vi "AcqType.vi"(11 "Ch & spans + mod limits":T2[](array[typedef]) {"low limit (-10V)" format="%.3f"; "high limit (10V)" format="%.3f"}) -> (0 "cDAQ i":i32[](array[numeric]), 1 "eDAQ i":i32[][](array[numeric]), 2 "cDAQ tasks":refnum<k21>[](array[refnum]), 3 "eDAQ tasks":refnum<k21>[](array[refnum]), 4 "PXI i":i32[](array[numeric]), 5 "PXIs":refnum<k21>[](array[refnum]))   [LabVIEW 2013]
doc: "Figures out if the channels requested are cDAQ, eDAQ or PXI and whether eDAQ channels are over multiple chassis.\n\n#optimation"
uses:
  Controls/Ch_and_Spans.ctl
  Channels_and_Index.ctl
panel:
  out "cDAQs":T1[][](array[typedef])
  out "PXI":T1[](array[typedef])
  out "Number of cDAQs":i32
  out "eDAQs":T1[][](array[typedef])
  out "Number of eDAQs":i32
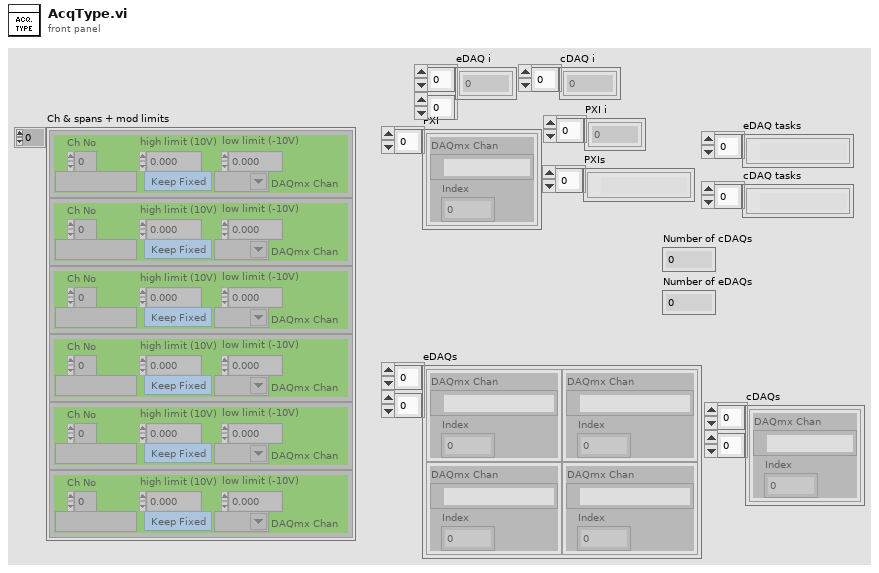
[diagram p1: front panel]
types:
  T1 = typedef "Channels_and_Index.ctl" = cluster{"DAQmx Chan":tag, "Index":i32}
  T2 = typedef "Ch_and_Spans.ctl" = cluster{"high limit (10V)":sgl, "low limit (-10V)":sgl, "Ch No":i16, "Var name":string, "Use Latest Calib":bool, "DAQmx Chan":tag}
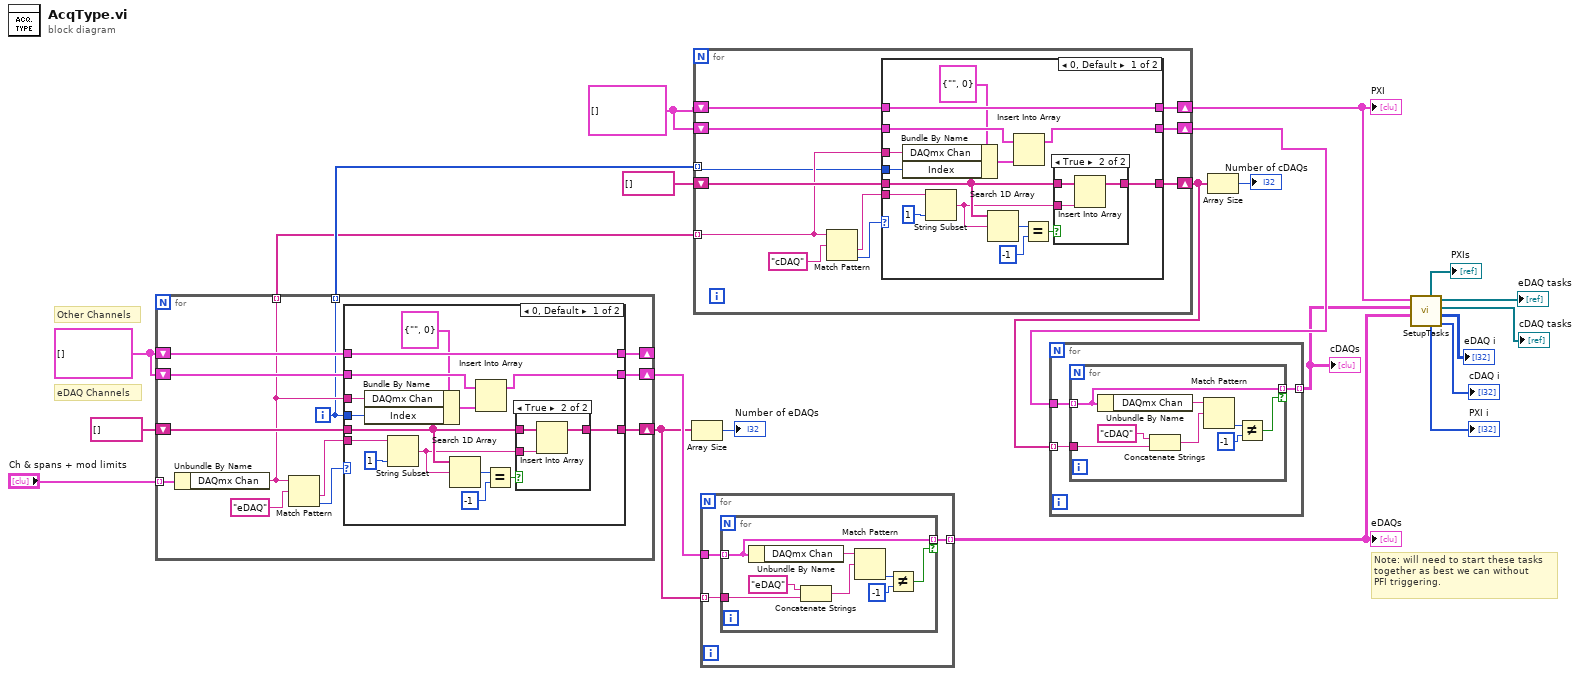
[diagram p0: block diagram]
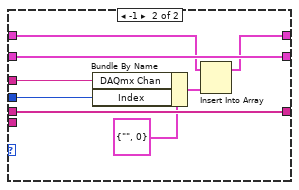
[diagram p3: hidden frame]
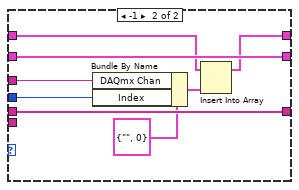
[diagram p5: hidden frame]
diagram:
  w15 = T1[] []
  w19 = T1[] []
  # "Note: will need to start these tasks \ntogether as best we can without\nPFI triggering."
  # "eDAQ Channels"
  # "Other Channels"
  n1 = for {
    tunnel: "Ch & spans + mod limits" -> [w34] mode=indexing
    shift-right: [w29] -> _
    shift-left: w19 -> [w31]
    shift-right: [w28] -> w18
    shift-left: w19 -> [w30]
    shift-right: [w25] -> w17
    shift-left: string[] [] -> [w27]
    tunnel: [w24] -> w3 mode=indexing
    tunnel: [w23] -> w4 mode=indexing
    i -> [w23]
    n2 = Unbundle By Name(w34) -> ("DAQmx Chan"=w24:tag)
    n3 = Match Pattern(string=w24, regular expression="eDAQ") -> (after substring=w26:string, offset past match=w32:i32)  [unwired: 1 in, 2 out]
    n4 = case shown="0, Default" w32 {
      tunnel: w24 -> [w36 w55]
      tunnel: w31 -> [w49 w60]
      tunnel: w30 -> [w48 w61]
      tunnel: [w49 w59] -> w29
      tunnel: [w47 w61] -> w28
      tunnel: w27 -> [w43 w58]
      tunnel: w26 -> [w45 _]
      tunnel: [w44 w58] -> w25
      tunnel: w23 -> [w35 w54]
      frame 0, Default {
        n5 = Bundle By Name(cluster=T1 {"DAQmx Chan"="", "Index"=0} ("Indexes"), "DAQmx Chan"=w36, "Index"=w35) -> (w37:T1)
        n6 = String Subset(string=w45, length (rest)=1 ("length (rest)")) -> (substring=w42:string)  [unwired: 1 in]
        n7 = Search 1D Array(1D array=w43, element=w42) -> (index of element=w41:i32)  [unwired: 1 in]
        n8 = Insert Into Array(array=w48, new element=w37) -> (w47:T1[])  [unwired: 1 in]
        n9 = Equal?(x=w41, y=-1) -> (x = y?=w39:bool)
        n10 = case shown="True" w39 {
          tunnel: [w50 w53] -> w44
          tunnel: w43 -> [w50 w52]
          tunnel: w42 -> [_ w51]
          frame False {
          }
          frame True {
            n11 = Insert Into Array(array=w52, new element=w51) -> (w53:string[])  [unwired: 1 in]
          }
        }
      }
      frame -1 {
        n12 = Bundle By Name(cluster=T1 {"DAQmx Chan"="", "Index"=0} ("Indexes"), "DAQmx Chan"=w55, "Index"=w54) -> (w56:T1)
        n13 = Insert Into Array(array=w60, new element=w56) -> (w59:T1[])  [unwired: 1 in]
      }
    }
  }
  n14 = Array Size(array=w17) -> (size(s)=→"Number of eDAQs":i32)
  n15 = for {
    shift-right: [w68] -> w13
    shift-left: w15 -> [w70]
    shift-right: [w67] -> w8
    shift-left: w15 -> [w69]
    shift-right: [w64] -> w9
    shift-left: string[] [] -> [w66]
    tunnel: w4 -> [w62] mode=indexing
    tunnel: w3 -> [w63] mode=indexing
    n16 = Match Pattern(string=w63, regular expression="cDAQ") -> (after substring=w65:string, offset past match=w71:i32)  [unwired: 1 in, 2 out]
    n17 = case shown="0, Default" w71 {
      tunnel: w63 -> [w74 w93]
      tunnel: w70 -> [w87 w98]
      tunnel: w69 -> [w86 w99]
      tunnel: [w87 w97] -> w68
      tunnel: [w85 w99] -> w67
      tunnel: w66 -> [w81 w96]
      tunnel: w65 -> [w83 _]
      tunnel: [w82 w96] -> w64
      tunnel: w62 -> [w73 w92]
      frame 0, Default {
        n18 = Bundle By Name(cluster=T1 {"DAQmx Chan"="", "Index"=0} ("Indexes"), "DAQmx Chan"=w74, "Index"=w73) -> (w75:T1)
        n19 = String Subset(string=w83, length (rest)=1 ("length (rest)")) -> (substring=w80:string)  [unwired: 1 in]
        n20 = Search 1D Array(1D array=w81, element=w80) -> (index of element=w79:i32)  [unwired: 1 in]
        n21 = Insert Into Array(array=w86, new element=w75) -> (w85:T1[])  [unwired: 1 in]
        n22 = Equal?(x=w79, y=-1) -> (x = y?=w77:bool)
        n23 = case shown="True" w77 {
          tunnel: [w88 w91] -> w82
          tunnel: w81 -> [w88 w90]
          tunnel: w80 -> [_ w89]
          frame False {
          }
          frame True {
            n24 = Insert Into Array(array=w90, new element=w89) -> (w91:string[])  [unwired: 1 in]
          }
        }
      }
      frame -1 {
        n25 = Bundle By Name(cluster=T1 {"DAQmx Chan"="", "Index"=0} ("Indexes"), "DAQmx Chan"=w93, "Index"=w92) -> (w94:T1)
        n26 = Insert Into Array(array=w98, new element=w94) -> (w97:T1[])  [unwired: 1 in]
      }
    }
  }
  "PXI" <- w13
  n27 = for {
    tunnel: w18 -> [w102]
    tunnel: w17 -> [w101] mode=indexing
    tunnel: [w100] -> w12 mode=indexing
    n28 = for {
      tunnel: w102 -> [w106] mode=indexing
      tunnel: w101 -> [w109]
      tunnel: [w106] -> w100 mode=indexing if=w104
      n29 = Unbundle By Name(w106) -> ("DAQmx Chan"=w107:tag)
      n30 = Concatenate Strings("eDAQ" ("regular expression"), w109) -> (w108:string)
      n31 = Match Pattern(string=w107, regular expression=w108) -> (offset past match=w105:i32)  [unwired: 1 in, 3 out]
      n32 = Not Equal?(x=w105, y=-1) -> (x != y?=w104:bool)
    }
  }
  "eDAQs" <- w12
  n33 = for {
    tunnel: w8 -> [w113]
    tunnel: w9 -> [w112] mode=indexing
    tunnel: [w111] -> w7 mode=indexing
    n34 = for {
      tunnel: w113 -> [w117] mode=indexing
      tunnel: w112 -> [w120]
      tunnel: [w117] -> w111 mode=indexing if=w115
      n35 = Unbundle By Name(w117) -> ("DAQmx Chan"=w118:tag)
      n36 = Concatenate Strings("cDAQ" ("regular expression"), w120) -> (w119:string)
      n37 = Match Pattern(string=w118, regular expression=w119) -> (offset past match=w116:i32)  [unwired: 1 in, 3 out]
      n38 = Not Equal?(x=w116, y=-1) -> (x != y?=w115:bool)
    }
  }
  "cDAQs" <- w7
  n39 = Array Size(array=w9) -> (size(s)=→"Number of cDAQs":i32)
  n40 = call "SetupTasks.vi"("eDAQs"=w12, "cDAQs"=w7, "PXI"=w13) -> ("cDAQ i"=→"cDAQ i":i32[], "eDAQ i"=→"eDAQ i":i32[][], "cDAQs"=→"cDAQ tasks":refnum<k21>[], "eDAQs"=→"eDAQ tasks":refnum<k21>[], "PXI i"=→"PXI i":i32[], "PXIs"=→"PXIs":refnum<k21>[])  [unwired: 3 in]
